vi "Simulacion_Teclas.vi"(11 "Numeric":i32=32) -> ()   [LabVIEW 2024]
doc: "Este VI se ecarga de simular una entrada del teclado con uso de librerias dinámicas (udll32).\n\nAutores: \nIvan Nieto Guerrero, David Alejandro Zarazúa Martínez.\n06/May/2025"
uses:
  user32.dll
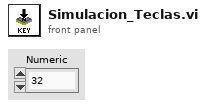
[diagram p1: front panel]
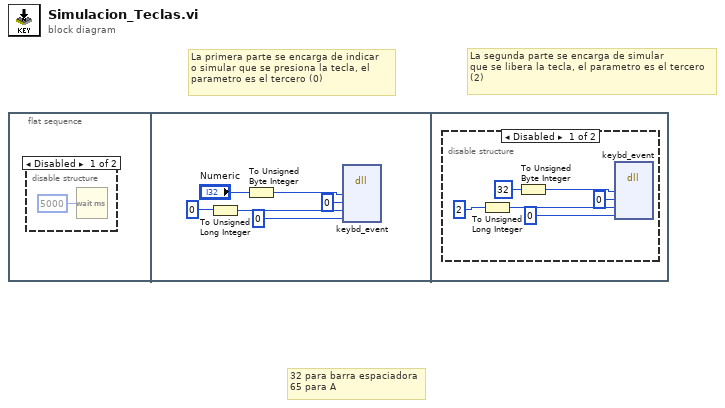
[diagram p0: block diagram]
diagram:
  # "32 para barra espaciadora\n65 para A"
  # "La segunda parte se encarga de simular\nque se libera la tecla, el parametro es el tercero\n(2)"
  # "La primera parte se encarga de indicar \no simular que se presiona la tecla, el \nparametro es el tercero (0)"
  n1 = flat-sequence {
    frame #0 {
      n2 = disable-structure shown="Disabled" {
        frame Disabled {
          n3 = Wait (ms)(milliseconds to wait=u32 5000) -> ()  [unwired: 1 out]
        }
        frame Enabled {
        }
      }
    }
    frame #1 {
      n4 = To Unsigned Long Integer(number=0) -> (unsigned 32bit integer=w2:u32)
      n5 = To Unsigned Byte Integer(number="Numeric") -> (unsigned 8bit integer=w4:u8)
      n6 = dll-call lib="user32.dll" fn="keybd_event"("bVk"=w4, "bScan"=u8 0, "dwFlags"=w2, "dwExtraInfo"=u32 0) -> ()  [unwired: 8 in, 2 out]
    }
    frame #2 {
      n7 = disable-structure shown="Disabled" {
        frame Disabled {
          n8 = To Unsigned Long Integer(number=2) -> (unsigned 32bit integer=w13:u32)
          n9 = To Unsigned Byte Integer(number=32) -> (unsigned 8bit integer=w11:u8)
          n10 = dll-call lib="user32.dll" fn="keybd_event"("bVk"=w11, "bScan"=u8 0, "dwFlags"=w13, "dwExtraInfo"=u32 0) -> ()  [unwired: 8 in, 2 out]
        }
        frame Enabled {
        }
      }
    }
  }
